vi "Read Meter Max.vi"(8 "error in (no error)":errorcluster, 11 "VISA resource name":refnum<visa-resource-name>) -> (0 "error out":errorcluster, 1 "Real Current":dbl, 2 "Total Current":dbl, 3 "VISA resource name out":refnum<visa-resource-name>)   [LabVIEW 2020, in "Associated Research 78XX Series.lvlib"]
doc: "RDM?\n\nThe instrument records the highest current reading during the test.\n\nAC: Returns two current readings, \"Total,Real\". Readings are in mA.\nDC: Returns one current reading. Readings are in uA."
uses:
  <instrlib>/Associated Research 78XX Series/Associated Research 78XX Series.lvlib
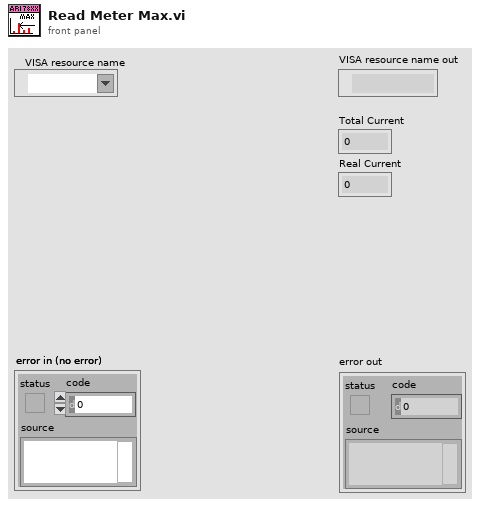
[diagram p1: front panel]
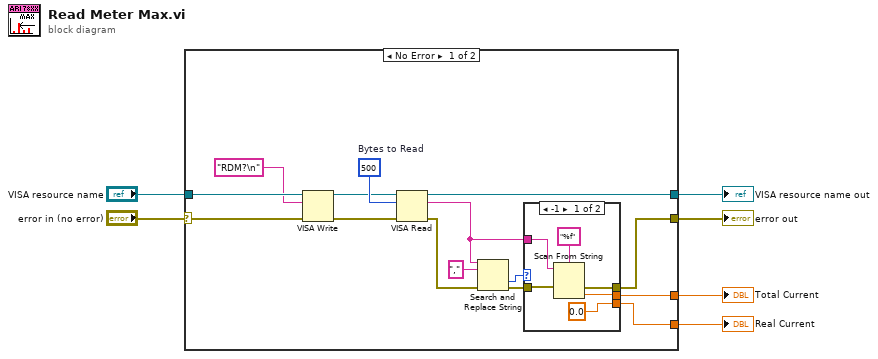
[diagram p0: block diagram]
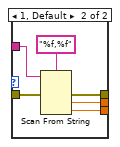
[diagram p2: hidden frame]
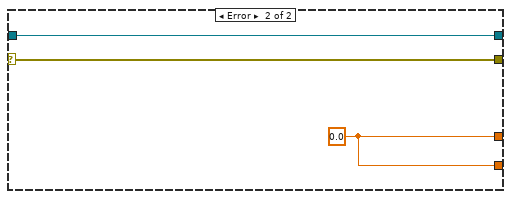
[diagram p3: hidden frame]
diagram:
  n1 = case shown="No Error" "error in (no error)" {
    selector: "error in (no error)" -> [w21 w36]
    tunnel: [w12 w36] -> w5
    tunnel: [w19 w35] -> w3
    tunnel: "VISA resource name" -> [w20 w35]
    tunnel: [w14 w34] -> w2
    tunnel: [w13 w34] -> w1
    frame No Error {
      w18 = u32 500  # Bytes to Read
      n2 = VISA Write(VISA resource name=w20, write buffer="RDM?\n" ("string (\"\")"), error in (no error)=w21) -> (VISA resource name out=w16:refnum<visa-resource-name>, error out=w17:errorcluster)  [unwired: 1 out]
      n3 = VISA Read(VISA resource name=w16, byte count=w18, error in (no error)=w17) -> (VISA resource name out=w19:refnum<visa-resource-name>, read buffer=w8:string, error out=w10:errorcluster)  [unwired: 1 out]
      n4 = Search and Replace String(input string=w8, search string=",", error in=w10) -> (offset past replacement=w7:i32, error out=w9:errorcluster)  [unwired: 5 in, 2 out]
      n5 = case shown="-1" w7 {
        tunnel: [w23 w32] -> w14
        tunnel: [0.0 w31] -> w13
        tunnel: [w24 w30] -> w12
        tunnel: w9 -> [w26 w29]
        tunnel: w8 -> [w25 w28]
        frame -1 {
          n6 = Scan From String(format string="%f", input string=w25, error in=w26) -> (error out=w24:errorcluster, output 1=w23:dbl)  [unwired: 2 in, 2 out]
        }
        frame 1, Default {
          n7 = Scan From String(format string="%f,%f", input string=w28, error in=w29) -> (error out=w30:errorcluster, output 1=w32:dbl, output 2=w31:dbl)  [unwired: 3 in, 2 out]
        }
      }
    }
    frame Error {
      w34 = 0.0
    }
  }
  "error out" <- w5
  "VISA resource name out" <- w3
  "Total Current" <- w2
  "Real Current" <- w1
